vi "Swerve Open 2020.vi"(10 "Drive Current Limit":dbl=50.0 format="%#_13g", 11 "Enum":T2(ring)) -> ()   [LabVIEW 2018]
uses:
  <vilib>/Rock Robotics/WPI/ThirdParty/Phoenix-LabVIEW/Motor Controller/Controls/CTRE_Phoenix_MotorControl_FeedbackDevice.ctl
  <vilib>/Rock Robotics/WPI/ThirdParty/Phoenix-LabVIEW/Motor Controller/Controls/CTRE_Phoenix_MotorControl_NeutralMode.ctl
  <vilib>/Rock Robotics/WPI/ThirdParty/Phoenix-LabVIEW/Motor Controller/Get/CTRE_Phoenix_MotorController_GetPulseWidthAll.vi
  <vilib>/Rock Robotics/Network Tables/NT Write Numeric Array.vi
  <vilib>/Rock Robotics/Network Tables/NT Read Numeric Array.vi
panel:
  out "Sticky Faults 12":T1
  out "Sticky Faults 11":T1={"Under Voltage"=TRUE, "Forward Limit Switch"=FALSE, "Reverse Limit Switch"=FALSE, "Forward Soft Limit"=FALSE, "Reverse Soft Limit"=FALSE, "Reset During Enable"=FALSE, "Sensor Overflow"=FALSE, "Sensor Out of Phase"=FALSE, "Hardware ESD Reset"=FALSE, "Remote Loss of Signal"=FALSE}
  out "Sticky Faults 10":T1
  out "Sticky Faults 9":T1
  in  "Offsets":dbl[](array[numeric])=[5398.0, 5987.0, 35324.0, 34409.0]
  in  "Constants":T3={"P"=6.0, "I"=0.0, "D"=60.0, "F"=1.0, "Max Vel"=900.0, "Max Accel"=3000.0}
  # "Little Swerve"
  # "8"
  # "6"
  # "1210"
  # "FL"
  # "1909"
  # "2531"
  # "0"
  # "0"
  # "FR"
  # "1604"
  # "BL"
  # "40"
  # "80"
  # "BR"
  # "0.806"
  # "1.23"
  # "900"
  # "900"
  # "3600"
  # "3600"
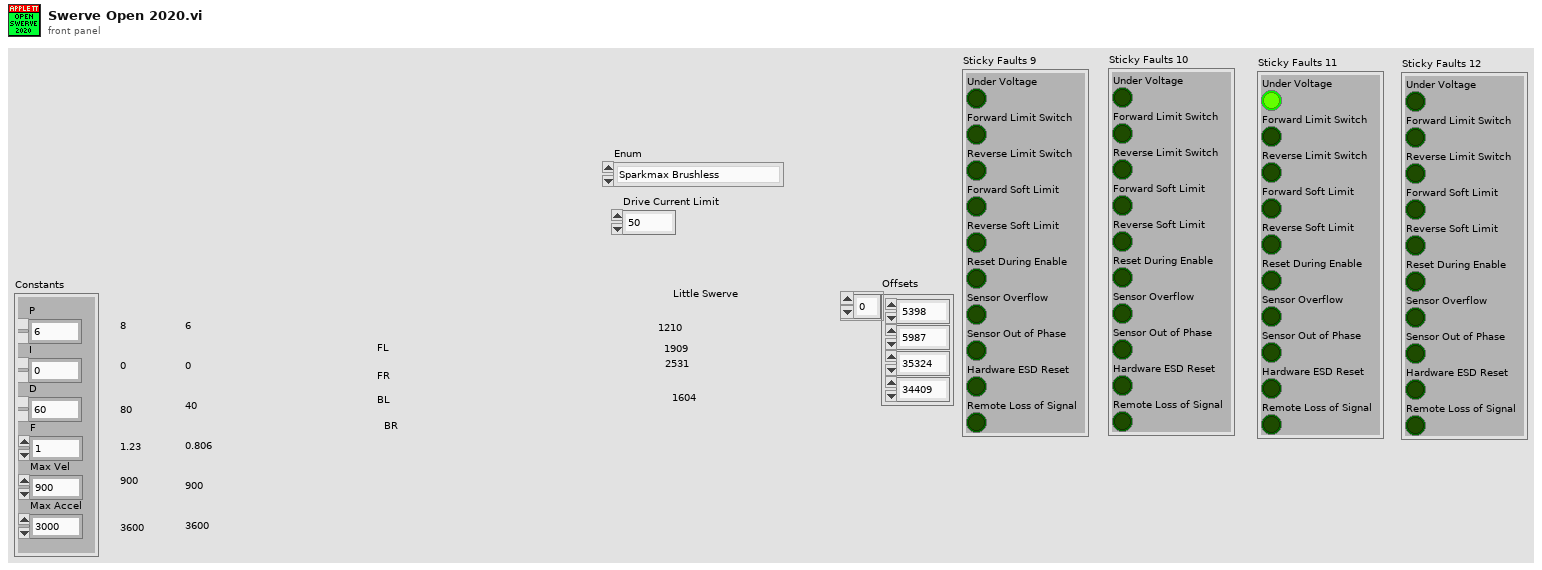
[diagram p1: front panel]
types:
  T1 = cluster{"Under Voltage":bool, "Forward Limit Switch":bool, "Reverse Limit Switch":bool, "Forward Soft Limit":bool, "Reverse Soft Limit":bool, "Reset During Enable":bool, "Sensor Overflow":bool, "Sensor Out of Phase":bool, "Hardware ESD Reset":bool, "Remote Loss of Signal":bool}
  T2 = enum16{"Sparkmax Brushless", "Talon SRX Brushed"}
  T3 = cluster{"P":dbl, "I":dbl, "D":dbl, "F":dbl, "Max Vel":dbl, "Max Accel":dbl}
  T4 = typedef "CTRE_Phoenix_MotorControl_NeutralMode.ctl" = enum8{"EEPROMSetting", "Override to Coast", "Override to Brake"}
  T5 = typedef "CTRE_Phoenix_MotorControl_FeedbackDevice.ctl" = i8
  T6 = typedef "WPI_MotorControlDeviceRef.ctl" = cluster{"DeviceStatus":errorcluster, "Type":T7, "PWM":cluster{"PWM Channel":T8, "DeadBand":T9}, "CAN":cluster{"Device Number":u8, "SetOutput VI Ref":variant, "GetOutput VI Ref":variant, "Enable VI Ref":variant, "Disable VI Ref":variant, "Data":variant}, "Invert":bool, "DIO PWM":cluster{"PWM \"Enable\" Channel":T8, "DIOChannel":T10, "PWM Rate":dbl}}
  T7 = typedef "WPI_MotorControlType.ctl" = enum16{"PWM", "CAN", "DIO PWM"}
  T8 = typedef "FPGA_DIOPWMChannel.ctl" = enum8{"PWM 0", "PWM 1", "PWM 2", "PWM 3", "PWM 4", "PWM 5", "PWM 6", "PWM 7", "PWM 8", "PWM 9", "PWM MXP 0", "PWM MXP 1", "PWM MXP 2", "PWM MXP 3", "PWM MXP 4", "PWM MXP 5", "PWM MXP 6", "PWM MXP 7", "PWM MXP 8", "PWM MXP 9", "Invalid"}
  T9 = typedef "WPI_PWMDeadband.ctl" = cluster{"Name":string, "maxPositivePwm":i32, "minPositivePwm":i32, "centerPwm":i32, "maxNegativePwm":i32, "minNegativePwm":i32, "angularRange":u16}
  T10 = typedef "FPGA_DIOChannel.ctl" = enum8{"DIO 0", "DIO 1", "DIO 2", "DIO 3", "DIO 4", "DIO 5", "DIO 6", "DIO 7", "DIO 8", "DIO 9", "DIO MXP 0", "DIO MXP 1", "DIO MXP 2", "DIO MXP 3", "DIO MXP 4", "DIO MXP 5", "DIO MXP 6", "DIO MXP 7", "DIO MXP 8", "DIO MXP 9", "DIO MXP 10", "DIO MXP 11", "DIO MXP 12", "DIO MXP 13", "DIO MXP 14", "DIO MXP 15", "SPI Port CS1", "SPI Port CS2", "SPI Port CS3", "SPI Port MISO", "SPI Port MOSI", "Invalid"}
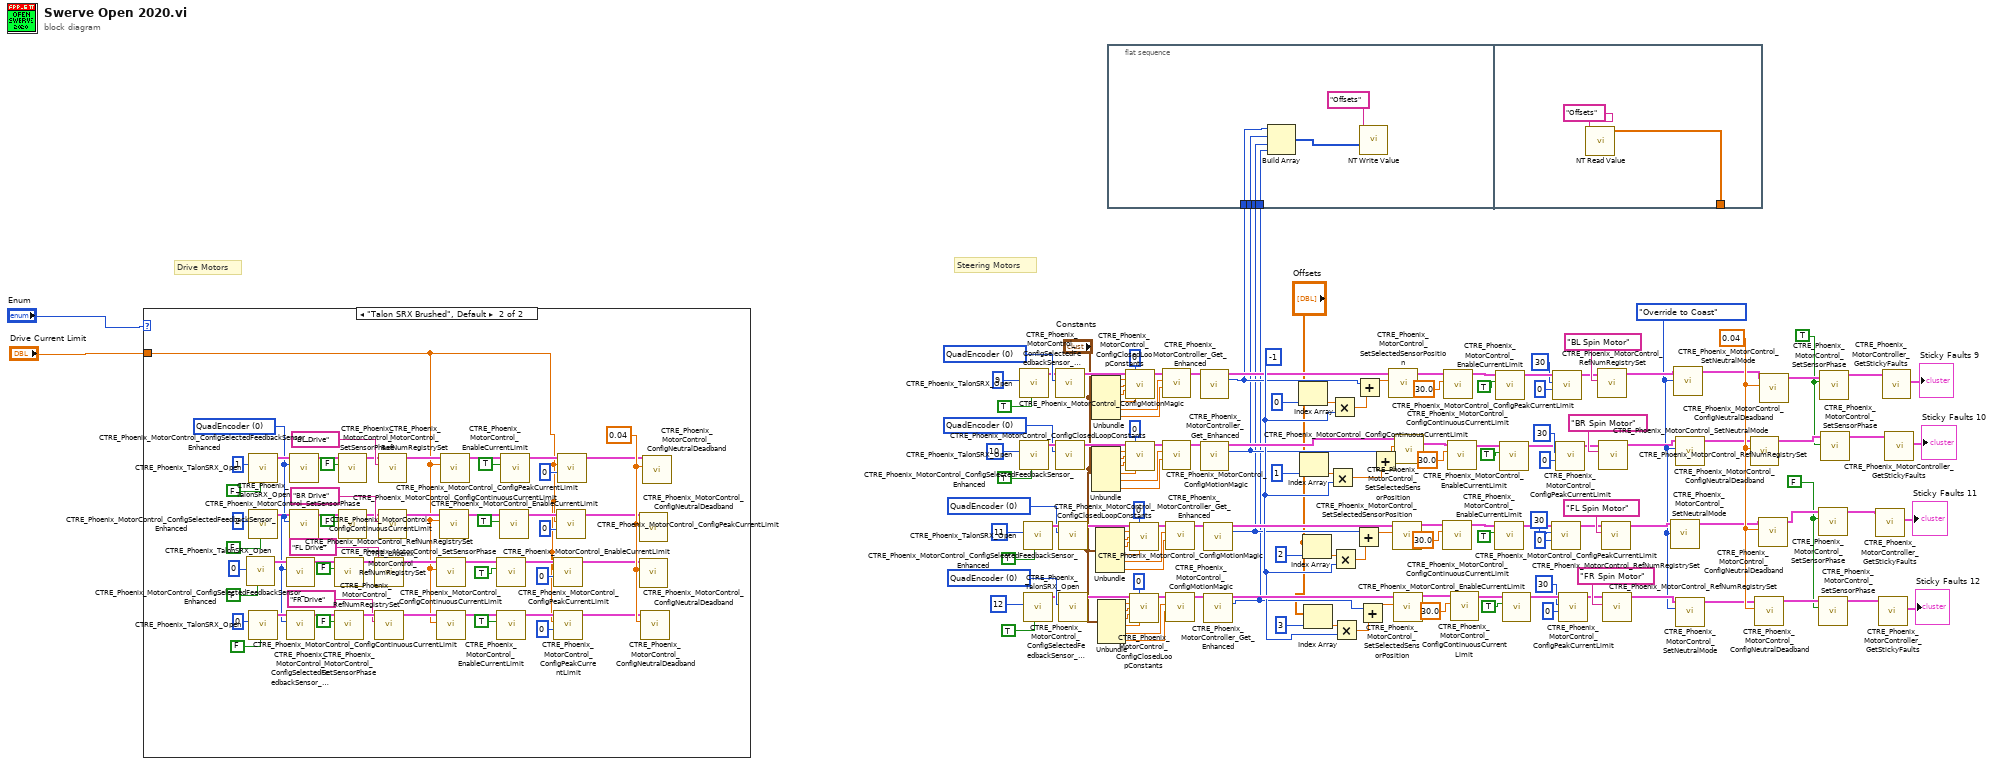
[diagram p0: block diagram]
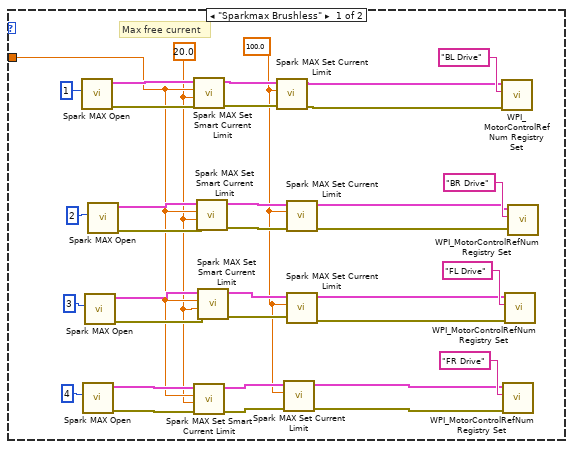
[diagram p2: hidden frame]
diagram:
  w10 = FALSE ("PhaseSensor")
  w11 = TRUE ("PhaseSensor")
  w32 = 0.04 ("Percent Deadband")
  w37 = CTRE_Phoenix_MotorControl_NeutralMode."Override to Coast" ("Motor Control Neutral Mode")
  w99 = T5 0 items=["None"=-1, "QuadEncoder"=0, "Analog"=2, "Tachometer"=4, "Pulse Width Encoded Position"=8, "Sensor Sum (S0 + S1)"=9, "Sensor Difference (D0 - D1)"=10, "Remote Source 0"=11, "Remote Source 1"=12, "Software Emulated"=15] ("Feedback Device")
  w100 = T5 0 items=["None"=-1, "QuadEncoder"=0, "Analog"=2, "Tachometer"=4, "Pulse Width Encoded Position"=8, "Sensor Sum (S0 + S1)"=9, "Sensor Difference (D0 - D1)"=10, "Remote Source 0"=11, "Remote Source 1"=12, "Software Emulated"=15] ("Feedback Device")
  w134 = T5 0 items=["None"=-1, "QuadEncoder"=0, "Analog"=2, "Tachometer"=4, "Pulse Width Encoded Position"=8, "Sensor Sum (S0 + S1)"=9, "Sensor Difference (D0 - D1)"=10, "Remote Source 0"=11, "Remote Source 1"=12, "Software Emulated"=15] ("Feedback Device")
  w133 = T5 0 items=["None"=-1, "QuadEncoder"=0, "Analog"=2, "Tachometer"=4, "Pulse Width Encoded Position"=8, "Sensor Sum (S0 + S1)"=9, "Sensor Difference (D0 - D1)"=10, "Remote Source 0"=11, "Remote Source 1"=12, "Software Emulated"=15] ("Feedback Device")
  w78 = -1 ("y")
  # "Steering Motors"
  # "Drive Motors"
  n1 = case shown="\"Talon SRX Brushed\", Default" "Enum" {
    tunnel: "Drive Current Limit" -> [w148 w181]
    frame "Sparkmax Brushless" {
      w146 = 20.0 ("Free Speed Current Limit (20A)")
      w147 = sgl 100.0 ("Current Limit A (100)")
      # "Max free current"
      n2 = call <vilib>:"Spark MAX Open.vi"("Device Number"=u8 1) -> ("error out"=w169:errorcluster, "MotorControlDeviceRef"=w168:T6)  [unwired: 9 in]
      n3 = call <vilib>:"Spark MAX Open.vi"("Device Number"=u8 4) -> ("error out"=w151:errorcluster, "MotorControlDeviceRef"=w152:T6)  [unwired: 9 in]
      n4 = call <vilib>:"Spark MAX Open.vi"("Device Number"=u8 3) -> ("error out"=w160:errorcluster, "MotorControlDeviceRef"=w161:T6)  [unwired: 9 in]
      n5 = call <vilib>:"Spark MAX Open.vi"("Device Number"=u8 2) -> ("error out"=w149:errorcluster, "MotorControlDeviceRef"=w150:T6)  [unwired: 9 in]
      n6 = call <vilib>:"Spark MAX Set Smart Current Limit.vi"("error in (no error)"=w169, "Free Speed Current Limit (20A)"=w146, "Primay Current Limit (80A)"=w148, "MotorControlDeviceRef in"=w168) -> ("error out"=w170:errorcluster, "MotorControlDeviceRef out"=w171:T6)  [unwired: 6 in]
      n7 = call <vilib>:"Spark MAX Set Smart Current Limit.vi"("error in (no error)"=w151, "Free Speed Current Limit (20A)"=w146, "Primay Current Limit (80A)"=w148, "MotorControlDeviceRef in"=w152) -> ("error out"=w162:errorcluster, "MotorControlDeviceRef out"=w163:T6)  [unwired: 6 in]
      n8 = call <vilib>:"Spark MAX Set Smart Current Limit.vi"("error in (no error)"=w149, "Free Speed Current Limit (20A)"=w146, "Primay Current Limit (80A)"=w148, "MotorControlDeviceRef in"=w150) -> ("error out"=w166:errorcluster, "MotorControlDeviceRef out"=w167:T6)  [unwired: 6 in]
      n9 = call <vilib>:"Spark MAX Set Smart Current Limit.vi"("error in (no error)"=w160, "Free Speed Current Limit (20A)"=w146, "Primay Current Limit (80A)"=w148, "MotorControlDeviceRef in"=w161) -> ("error out"=w164:errorcluster, "MotorControlDeviceRef out"=w165:T6)  [unwired: 6 in]
      n10 = call <vilib>:"Spark MAX Set Current Limit.vi"("error in (no error)"=w170, "Current Limit A (100)"=w147, "MotorControlDeviceRef in"=w171) -> ("error out"=w172:errorcluster, "MotorControlDeviceRef out"=w173:T6)  [unwired: 7 in]
      n11 = call <vilib>:"Spark MAX Set Current Limit.vi"("error in (no error)"=w162, "Current Limit A (100)"=w147, "MotorControlDeviceRef in"=w163) -> ("error out"=w153:errorcluster, "MotorControlDeviceRef out"=w154:T6)  [unwired: 7 in]
      n12 = call <vilib>:"Spark MAX Set Current Limit.vi"("error in (no error)"=w166, "Current Limit A (100)"=w147, "MotorControlDeviceRef in"=w167) -> ("error out"=w156:errorcluster, "MotorControlDeviceRef out"=w157:T6)  [unwired: 7 in]
      n13 = call <vilib>:"Spark MAX Set Current Limit.vi"("error in (no error)"=w164, "Current Limit A (100)"=w147, "MotorControlDeviceRef in"=w165) -> ("error out"=w158:errorcluster, "MotorControlDeviceRef out"=w159:T6)  [unwired: 7 in]
      n14 = call <vilib>:"WPI_MotorControlRefNum Registry Set.vi"("error in (no error)"=w172, "refnum name"="BL Drive", "MotorControlDevRef"=w173) -> ()  [unwired: 7 in, 2 out]
      n15 = call <vilib>:"WPI_MotorControlRefNum Registry Set.vi"("error in (no error)"=w153, "refnum name"="FR Drive", "MotorControlDevRef"=w154) -> ()  [unwired: 7 in, 2 out]
      n16 = call <vilib>:"WPI_MotorControlRefNum Registry Set.vi"("error in (no error)"=w158, "refnum name"="FL Drive", "MotorControlDevRef"=w159) -> ()  [unwired: 7 in, 2 out]
      n17 = call <vilib>:"WPI_MotorControlRefNum Registry Set.vi"("error in (no error)"=w156, "refnum name"="BR Drive", "MotorControlDevRef"=w157) -> ()  [unwired: 7 in, 2 out]
    }
    frame "Talon SRX Brushed", Default {
      w191 = 0.04 ("Percent Deadband")
      (unwired) u8 0 ("Device Number")
      (unwired) u8 0 ("Device Number")
      (unwired) u8 0 ("Device Number")
      (unwired) u8 0 ("Device Number")
      w192 = T5 0 items=["None"=-1, "QuadEncoder"=0, "Analog"=2, "Tachometer"=4, "Pulse Width Encoded Position"=8, "Sensor Sum (S0 + S1)"=9, "Sensor Difference (D0 - D1)"=10, "Remote Source 0"=11, "Remote Source 1"=12, "Software Emulated"=15] ("Feedback Device")
      n18 = call <vilib>:"CTRE_Phoenix_TalonSRX_Open.vi"("Invert"=FALSE, "Device Number"=u8 3) -> ("CAN Talon SRX Ref"=w199:T6)  [unwired: 8 in, 1 out]
      n19 = call <vilib>:"CTRE_Phoenix_TalonSRX_Open.vi"("Invert"=FALSE, "Device Number"=u8 1) -> ("CAN Talon SRX Ref"=w230:T6)  [unwired: 8 in, 1 out]
      n20 = call <vilib>:"CTRE_Phoenix_TalonSRX_Open.vi"("Invert"=FALSE, "Device Number"=u8 2) -> ("CAN Talon SRX Ref"=w231:T6)  [unwired: 8 in, 1 out]
      n21 = call <vilib>:"CTRE_Phoenix_TalonSRX_Open.vi"("Invert"=FALSE, "Device Number"=u8 4) -> ("CAN Talon SRX Ref"=w203:T6)  [unwired: 8 in, 1 out]
      n22 = call <vilib>:"CTRE_Phoenix_MotorControl_ConfigSelectedFeedbackSensor_Enhanced.vi"("Feedback Device"=w192, "PhoenixMotorControlDevRef"=w199) -> ("PhoenixMotorControlDevRef"=w198:T6)  [unwired: 8 in, 1 out]
      n23 = call <vilib>:"CTRE_Phoenix_MotorControl_ConfigSelectedFeedbackSensor_Enhanced.vi"("Feedback Device"=w192, "PhoenixMotorControlDevRef"=w203) -> ("PhoenixMotorControlDevRef"=w205:T6)  [unwired: 8 in, 1 out]
      n24 = call <vilib>:"CTRE_Phoenix_MotorControl_ConfigSelectedFeedbackSensor_Enhanced.vi"("Feedback Device"=w192, "PhoenixMotorControlDevRef"=w230) -> ("PhoenixMotorControlDevRef"=w226:T6)  [unwired: 8 in, 1 out]
      n25 = call <vilib>:"CTRE_Phoenix_MotorControl_ConfigSelectedFeedbackSensor_Enhanced.vi"("Feedback Device"=w192, "PhoenixMotorControlDevRef"=w231) -> ("PhoenixMotorControlDevRef"=w229:T6)  [unwired: 8 in, 1 out]
      n26 = call <vilib>:"CTRE_Phoenix_MotorControl_SetSensorPhase.vi"("PhaseSensor"=FALSE, "PhoenixMotorControlDevRef"=w198) -> ("PhoenixMotorControlDevRef"=w197:T6)  [unwired: 8 in, 1 out]
      n27 = call <vilib>:"CTRE_Phoenix_MotorControl_SetSensorPhase.vi"("PhaseSensor"=FALSE, "PhoenixMotorControlDevRef"=w205) -> ("PhoenixMotorControlDevRef"=w204:T6)  [unwired: 8 in, 1 out]
      n28 = call <vilib>:"CTRE_Phoenix_MotorControl_SetSensorPhase.vi"("PhaseSensor"=FALSE, "PhoenixMotorControlDevRef"=w226) -> ("PhoenixMotorControlDevRef"=w227:T6)  [unwired: 8 in, 1 out]
      n29 = call <vilib>:"CTRE_Phoenix_MotorControl_SetSensorPhase.vi"("PhaseSensor"=FALSE, "PhoenixMotorControlDevRef"=w229) -> ("PhoenixMotorControlDevRef"=w228:T6)  [unwired: 8 in, 1 out]
      n30 = call <vilib>:"CTRE_Phoenix_MotorControl_RefNumRegistrySet.vi"("refnum name"="FL Drive", "PhoenixMotorControlDevRef"=w197) -> ("PhoenixMotorControlDevRef"=w196:T6)  [unwired: 8 in, 1 out]
      n31 = call <vilib>:"CTRE_Phoenix_MotorControl_RefNumRegistrySet.vi"("refnum name"="FR Drive", "PhoenixMotorControlDevRef"=w204) -> ("PhoenixMotorControlDevRef"=w213:T6)  [unwired: 8 in, 1 out]
      n32 = call <vilib>:"CTRE_Phoenix_MotorControl_RefNumRegistrySet.vi"("refnum name"="BL Drive", "PhoenixMotorControlDevRef"=w227) -> ("PhoenixMotorControlDevRef"=w214:T6)  [unwired: 8 in, 1 out]
      n33 = call <vilib>:"CTRE_Phoenix_MotorControl_RefNumRegistrySet.vi"("refnum name"="BR Drive", "PhoenixMotorControlDevRef"=w228) -> ("PhoenixMotorControlDevRef"=w219:T6)  [unwired: 8 in, 1 out]
      n34 = call <vilib>:"CTRE_Phoenix_MotorControl_ConfigContinuousCurrentLimit.vi"("Continuous Current Limit (Amps)"=w181, "PhoenixMotorControlDevRef"=w196) -> ("PhoenixMotorControlDevRef"=w195:T6)  [unwired: 8 in, 1 out]
      n35 = call <vilib>:"CTRE_Phoenix_MotorControl_ConfigContinuousCurrentLimit.vi"("Continuous Current Limit (Amps)"=w181, "PhoenixMotorControlDevRef"=w213) -> ("PhoenixMotorControlDevRef"=w208:T6)  [unwired: 8 in, 1 out]
      n36 = call <vilib>:"CTRE_Phoenix_MotorControl_ConfigContinuousCurrentLimit.vi"("Continuous Current Limit (Amps)"=w181, "PhoenixMotorControlDevRef"=w219) -> ("PhoenixMotorControlDevRef"=w223:T6)  [unwired: 8 in, 1 out]
      n37 = call <vilib>:"CTRE_Phoenix_MotorControl_ConfigContinuousCurrentLimit.vi"("Continuous Current Limit (Amps)"=w181, "PhoenixMotorControlDevRef"=w214) -> ("PhoenixMotorControlDevRef"=w215:T6)  [unwired: 8 in, 1 out]
      n38 = call <vilib>:"CTRE_Phoenix_MotorControl_EnableCurrentLimit.vi"("Enable Current Limit?"=TRUE, "PhoenixMotorControlDevRef"=w195) -> ("PhoenixMotorControlDevRef"=w194:T6)  [unwired: 8 in, 1 out]
      n39 = call <vilib>:"CTRE_Phoenix_MotorControl_EnableCurrentLimit.vi"("Enable Current Limit?"=TRUE, "PhoenixMotorControlDevRef"=w208) -> ("PhoenixMotorControlDevRef"=w211:T6)  [unwired: 8 in, 1 out]
      n40 = call <vilib>:"CTRE_Phoenix_MotorControl_EnableCurrentLimit.vi"("Enable Current Limit?"=TRUE, "PhoenixMotorControlDevRef"=w223) -> ("PhoenixMotorControlDevRef"=w220:T6)  [unwired: 8 in, 1 out]
      n41 = call <vilib>:"CTRE_Phoenix_MotorControl_EnableCurrentLimit.vi"("Enable Current Limit?"=TRUE, "PhoenixMotorControlDevRef"=w215) -> ("PhoenixMotorControlDevRef"=w218:T6)  [unwired: 8 in, 1 out]
      n42 = call <vilib>:"CTRE_Phoenix_MotorControl_ConfigPeakCurrentLimit.vi"("Peak Current Maximum Duration (ms)"=0, "Peak Current (Amps)"=w181, "PhoenixMotorControlDevRef"=w194) -> ("PhoenixMotorControlDevRef"=w184:T6)  [unwired: 7 in, 1 out]
      n43 = call <vilib>:"CTRE_Phoenix_MotorControl_ConfigPeakCurrentLimit.vi"("Peak Current Maximum Duration (ms)"=0, "Peak Current (Amps)"=w181, "PhoenixMotorControlDevRef"=w211) -> ("PhoenixMotorControlDevRef"=w183:T6)  [unwired: 7 in, 1 out]
      n44 = call <vilib>:"CTRE_Phoenix_MotorControl_ConfigPeakCurrentLimit.vi"("Peak Current Maximum Duration (ms)"=0, "Peak Current (Amps)"=w181, "PhoenixMotorControlDevRef"=w220) -> ("PhoenixMotorControlDevRef"=w185:T6)  [unwired: 7 in, 1 out]
      n45 = call <vilib>:"CTRE_Phoenix_MotorControl_ConfigPeakCurrentLimit.vi"("Peak Current Maximum Duration (ms)"=0, "Peak Current (Amps)"=w181, "PhoenixMotorControlDevRef"=w218) -> ("PhoenixMotorControlDevRef"=w186:T6)  [unwired: 7 in, 1 out]
      n46 = call <vilib>:"CTRE_Phoenix_MotorControl_ConfigNeutralDeadband.vi"("Percent Deadband"=w191, "PhoenixMotorControlDevRef"=w185) -> ()  [unwired: 8 in, 2 out]
      n47 = call <vilib>:"CTRE_Phoenix_MotorControl_ConfigNeutralDeadband.vi"("Percent Deadband"=w191, "PhoenixMotorControlDevRef"=w184) -> ()  [unwired: 8 in, 2 out]
      n48 = call <vilib>:"CTRE_Phoenix_MotorControl_ConfigNeutralDeadband.vi"("Percent Deadband"=w191, "PhoenixMotorControlDevRef"=w183) -> ()  [unwired: 8 in, 2 out]
      n49 = call <vilib>:"CTRE_Phoenix_MotorControl_ConfigNeutralDeadband.vi"("Percent Deadband"=w191, "PhoenixMotorControlDevRef"=w186) -> ()  [unwired: 8 in, 2 out]
    }
  }
  n50 = call <vilib>:"CTRE_Phoenix_TalonSRX_Open.vi"("Invert"=TRUE, "Device Number"=u8 9) -> ("CAN Talon SRX Ref"=w123:T6)  [unwired: 8 in, 1 out]
  n51 = call <vilib>:"CTRE_Phoenix_TalonSRX_Open.vi"("Invert"=TRUE, "Device Number"=u8 10) -> ("CAN Talon SRX Ref"=w143:T6)  [unwired: 8 in, 1 out]
  n52 = call <vilib>:"CTRE_Phoenix_TalonSRX_Open.vi"("Invert"=TRUE, "Device Number"=u8 11) -> ("CAN Talon SRX Ref"=w110:T6)  [unwired: 8 in, 1 out]
  n53 = call <vilib>:"CTRE_Phoenix_TalonSRX_Open.vi"("Invert"=TRUE, "Device Number"=u8 12) -> ("CAN Talon SRX Ref"=w91:T6)  [unwired: 8 in, 1 out]
  n54 = call <vilib>:"CTRE_Phoenix_MotorControl_ConfigSelectedFeedbackSensor_Enhanced.vi"("Feedback Device"=w133, "PhoenixMotorControlDevRef"=w123) -> ("PhoenixMotorControlDevRef"=w126:T6)  [unwired: 8 in, 1 out]
  n55 = call <vilib>:"CTRE_Phoenix_MotorControl_ConfigSelectedFeedbackSensor_Enhanced.vi"("Feedback Device"=w134, "PhoenixMotorControlDevRef"=w143) -> ("PhoenixMotorControlDevRef"=w141:T6)  [unwired: 8 in, 1 out]
  n56 = call <vilib>:"CTRE_Phoenix_MotorControl_ConfigSelectedFeedbackSensor_Enhanced.vi"("Feedback Device"=w100, "PhoenixMotorControlDevRef"=w110) -> ("PhoenixMotorControlDevRef"=w107:T6)  [unwired: 8 in, 1 out]
  n57 = call <vilib>:"CTRE_Phoenix_MotorControl_ConfigSelectedFeedbackSensor_Enhanced.vi"("Feedback Device"=w99, "PhoenixMotorControlDevRef"=w91) -> ("PhoenixMotorControlDevRef"=w94:T6)  [unwired: 8 in, 1 out]
  n58 = Unbundle("Constants") -> ("P"=w127:dbl, "I"=w128:dbl, "D"=w129:dbl, "F"=w130:dbl, "Max Vel"=w131:dbl, "Max Accel"=w132:dbl)
  n59 = Unbundle("Constants") -> ("P"=w140:dbl, "I"=w139:dbl, "D"=w138:dbl, "F"=w137:dbl, "Max Vel"=w136:dbl, "Max Accel"=w135:dbl)
  n60 = Unbundle("Constants") -> ("P"=w106:dbl, "I"=w105:dbl, "D"=w104:dbl, "F"=w103:dbl, "Max Vel"=w102:dbl, "Max Accel"=w101:dbl)
  n61 = Unbundle("Constants") -> ("P"=w95:dbl, "I"=w96:dbl, "D"=w97:dbl, "F"=w98:dbl, "Max Vel"=w77:dbl, "Max Accel"=w76:dbl)
  n62 = flat-sequence {
    tunnel: w15 -> [w241]
    tunnel: w14 -> [w240]
    tunnel: w13 -> [w239]
    tunnel: w12 -> [w238]
    tunnel: [w242] -> _
    frame #0 {
      n63 = Build Array(w241, w240, w239, w238) -> (w236:i32[])
      n64 = call-poly <vilib>:"NT Write Value.vi"("Numeric Array"=w236, "Name"="Offsets") -> ()  [unwired: 9 in, 1 out]
    }
    frame #1 {
      n65 = call-poly <vilib>:"NT Read Value.vi"("Name"="Offsets") -> ("Numeric Array"=w242:dbl[])  [unwired: 9 in, 1 out]
    }
  }
  n66 = call <vilib>:"CTRE_Phoenix_MotorControl_ConfigClosedLoopConstants.vi"("PhoenixMotorControlDevRef"=w126, "slotIdx"=0, "P"=w127, "I"=w128, "D"=w129, "F"=w130) -> ("PhoenixMotorControlDevRef"=w125:T6)  [unwired: 8 in, 1 out]
  n67 = call <vilib>:"CTRE_Phoenix_MotorControl_ConfigClosedLoopConstants.vi"("PhoenixMotorControlDevRef"=w141, "slotIdx"=0, "P"=w140, "I"=w139, "D"=w138, "F"=w137) -> ("PhoenixMotorControlDevRef"=w142:T6)  [unwired: 8 in, 1 out]
  n68 = call <vilib>:"CTRE_Phoenix_MotorControl_ConfigClosedLoopConstants.vi"("PhoenixMotorControlDevRef"=w107, "slotIdx"=0, "P"=w106, "I"=w105, "D"=w104, "F"=w103) -> ("PhoenixMotorControlDevRef"=w108:T6)  [unwired: 8 in, 1 out]
  n69 = call <vilib>:"CTRE_Phoenix_MotorControl_ConfigClosedLoopConstants.vi"("PhoenixMotorControlDevRef"=w94, "slotIdx"=0, "P"=w95, "I"=w96, "D"=w97, "F"=w98) -> ("PhoenixMotorControlDevRef"=w93:T6)  [unwired: 8 in, 1 out]
  n70 = call <vilib>:"CTRE_Phoenix_MotorControl_ConfigMotionMagic.vi"("Acceleration"=w132, "Cruise Velocity"=w131, "PhoenixMotorControlDevRef"=w125) -> ("PhoenixMotorControlDevRef"=w124:T6)  [unwired: 7 in, 1 out]
  n71 = call <vilib>:"CTRE_Phoenix_MotorControl_ConfigMotionMagic.vi"("Acceleration"=w135, "Cruise Velocity"=w136, "PhoenixMotorControlDevRef"=w142) -> ("PhoenixMotorControlDevRef"=w111:T6)  [unwired: 7 in, 1 out]
  n72 = call <vilib>:"CTRE_Phoenix_MotorControl_ConfigMotionMagic.vi"("Acceleration"=w101, "Cruise Velocity"=w102, "PhoenixMotorControlDevRef"=w108) -> ("PhoenixMotorControlDevRef"=w109:T6)  [unwired: 7 in, 1 out]
  n73 = call <vilib>:"CTRE_Phoenix_MotorControl_ConfigMotionMagic.vi"("Acceleration"=w76, "Cruise Velocity"=w77, "PhoenixMotorControlDevRef"=w93) -> ("PhoenixMotorControlDevRef"=w92:T6)  [unwired: 7 in, 1 out]
  n74 = call-poly <vilib>:"CTRE_Phoenix_MotorController_Get_Enhanced.vi"("PhoenixMotorControlDevRef"=w124) -> ("PhoenixMotorControlDevRef"=w16:T6, "Pulse Width Position"=w15:i32)  [unwired: 9 in, 4 out]
  n75 = call-poly <vilib>:"CTRE_Phoenix_MotorController_Get_Enhanced.vi"("PhoenixMotorControlDevRef"=w111) -> ("PhoenixMotorControlDevRef"=w114:T6, "Pulse Width Position"=w14:i32)  [unwired: 9 in, 4 out]
  n76 = call-poly <vilib>:"CTRE_Phoenix_MotorController_Get_Enhanced.vi"("PhoenixMotorControlDevRef"=w109) -> ("PhoenixMotorControlDevRef"=w82:T6, "Pulse Width Position"=w13:i32)  [unwired: 9 in, 4 out]
  n77 = call-poly <vilib>:"CTRE_Phoenix_MotorController_Get_Enhanced.vi"("PhoenixMotorControlDevRef"=w92) -> ("PhoenixMotorControlDevRef"=w85:T6, "Pulse Width Position"=w12:i32)  [unwired: 9 in, 4 out]
  n78 = Index Array(array="Offsets", index=0) -> (element=w36:dbl)
  n79 = Index Array(array="Offsets", index=1) -> (element=w35:dbl)
  n80 = Index Array(array="Offsets", index=2) -> (element=w34:dbl)
  n81 = Index Array(array="Offsets", index=3) -> (element=w33:dbl)
  n82 = Multiply(x=w35, y=w78) -> (x*y=w115:dbl)
  n83 = Multiply(x=w36, y=w78) -> (x*y=w21:dbl)
  n84 = Multiply(x=w34, y=w78) -> (x*y=w22:dbl)
  n85 = Multiply(x=w33, y=w78) -> (x*y=w23:dbl)
  n86 = Add(x=w13, y=w22) -> (x+y=w18:dbl)
  n87 = Add(x=w15, y=w21) -> (x+y=w20:dbl)
  n88 = Add(x=w12, y=w23) -> (x+y=w17:dbl)
  n89 = Add(x=w14, y=w115) -> (x+y=w19:dbl)
  n90 = call <vilib>:"CTRE_Phoenix_MotorControl_SetSelectedSensorPosition.vi"("New Sensor Position"=w20, "PhoenixMotorControlDevRef"=w16) -> ("PhoenixMotorControlDevRef"=w51:T6)  [unwired: 8 in, 1 out]
  n91 = call <vilib>:"CTRE_Phoenix_MotorControl_SetSelectedSensorPosition.vi"("New Sensor Position"=w18, "PhoenixMotorControlDevRef"=w82) -> ("PhoenixMotorControlDevRef"=w47:T6)  [unwired: 8 in, 1 out]
  n92 = call <vilib>:"CTRE_Phoenix_MotorControl_SetSelectedSensorPosition.vi"("New Sensor Position"=w17, "PhoenixMotorControlDevRef"=w85) -> ("PhoenixMotorControlDevRef"=w48:T6)  [unwired: 8 in, 1 out]
  n93 = call <vilib>:"CTRE_Phoenix_MotorControl_SetSelectedSensorPosition.vi"("New Sensor Position"=w19, "PhoenixMotorControlDevRef"=w114) -> ("PhoenixMotorControlDevRef"=w50:T6)  [unwired: 8 in, 1 out]
  n94 = call <vilib>:"CTRE_Phoenix_MotorControl_ConfigContinuousCurrentLimit.vi"("Continuous Current Limit (Amps)"=30.0, "PhoenixMotorControlDevRef"=w47) -> ("PhoenixMotorControlDevRef"=w54:T6)  [unwired: 8 in, 1 out]
  n95 = call <vilib>:"CTRE_Phoenix_MotorControl_ConfigContinuousCurrentLimit.vi"("Continuous Current Limit (Amps)"=30.0, "PhoenixMotorControlDevRef"=w51) -> ("PhoenixMotorControlDevRef"=w65:T6)  [unwired: 8 in, 1 out]
  n96 = call <vilib>:"CTRE_Phoenix_MotorControl_ConfigContinuousCurrentLimit.vi"("Continuous Current Limit (Amps)"=30.0, "PhoenixMotorControlDevRef"=w50) -> ("PhoenixMotorControlDevRef"=w74:T6)  [unwired: 8 in, 1 out]
  n97 = call <vilib>:"CTRE_Phoenix_MotorControl_ConfigContinuousCurrentLimit.vi"("Continuous Current Limit (Amps)"=30.0, "PhoenixMotorControlDevRef"=w48) -> ("PhoenixMotorControlDevRef"=w56:T6)  [unwired: 8 in, 1 out]
  n98 = call <vilib>:"CTRE_Phoenix_MotorControl_EnableCurrentLimit.vi"("Enable Current Limit?"=TRUE, "PhoenixMotorControlDevRef"=w54) -> ("PhoenixMotorControlDevRef"=w53:T6)  [unwired: 8 in, 1 out]
  n99 = call <vilib>:"CTRE_Phoenix_MotorControl_EnableCurrentLimit.vi"("Enable Current Limit?"=TRUE, "PhoenixMotorControlDevRef"=w65) -> ("PhoenixMotorControlDevRef"=w69:T6)  [unwired: 8 in, 1 out]
  n100 = call <vilib>:"CTRE_Phoenix_MotorControl_EnableCurrentLimit.vi"("Enable Current Limit?"=TRUE, "PhoenixMotorControlDevRef"=w74) -> ("PhoenixMotorControlDevRef"=w70:T6)  [unwired: 8 in, 1 out]
  n101 = call <vilib>:"CTRE_Phoenix_MotorControl_EnableCurrentLimit.vi"("Enable Current Limit?"=TRUE, "PhoenixMotorControlDevRef"=w56) -> ("PhoenixMotorControlDevRef"=w60:T6)  [unwired: 8 in, 1 out]
  n102 = call <vilib>:"CTRE_Phoenix_MotorControl_ConfigPeakCurrentLimit.vi"("Peak Current Maximum Duration (ms)"=0, "Peak Current (Amps)"=30, "PhoenixMotorControlDevRef"=w53) -> ("PhoenixMotorControlDevRef"=w43:T6)  [unwired: 7 in, 1 out]
  n103 = call <vilib>:"CTRE_Phoenix_MotorControl_ConfigPeakCurrentLimit.vi"("Peak Current Maximum Duration (ms)"=0, "Peak Current (Amps)"=30, "PhoenixMotorControlDevRef"=w69) -> ("PhoenixMotorControlDevRef"=w45:T6)  [unwired: 7 in, 1 out]
  n104 = call <vilib>:"CTRE_Phoenix_MotorControl_ConfigPeakCurrentLimit.vi"("Peak Current Maximum Duration (ms)"=0, "Peak Current (Amps)"=30, "PhoenixMotorControlDevRef"=w70) -> ("PhoenixMotorControlDevRef"=w44:T6)  [unwired: 7 in, 1 out]
  n105 = call <vilib>:"CTRE_Phoenix_MotorControl_ConfigPeakCurrentLimit.vi"("Peak Current Maximum Duration (ms)"=0, "Peak Current (Amps)"=30, "PhoenixMotorControlDevRef"=w60) -> ("PhoenixMotorControlDevRef"=w42:T6)  [unwired: 7 in, 1 out]
  n106 = call <vilib>:"CTRE_Phoenix_MotorControl_RefNumRegistrySet.vi"("refnum name"="BL Spin Motor", "PhoenixMotorControlDevRef"=w45) -> ("PhoenixMotorControlDevRef"=w41:T6)  [unwired: 8 in, 1 out]
  n107 = call <vilib>:"CTRE_Phoenix_MotorControl_RefNumRegistrySet.vi"("refnum name"="BR Spin Motor", "PhoenixMotorControlDevRef"=w44) -> ("PhoenixMotorControlDevRef"=w40:T6)  [unwired: 8 in, 1 out]
  n108 = call <vilib>:"CTRE_Phoenix_MotorControl_RefNumRegistrySet.vi"("refnum name"="FL Spin Motor", "PhoenixMotorControlDevRef"=w43) -> ("PhoenixMotorControlDevRef"=w39:T6)  [unwired: 8 in, 1 out]
  n109 = call <vilib>:"CTRE_Phoenix_MotorControl_RefNumRegistrySet.vi"("refnum name"="FR Spin Motor", "PhoenixMotorControlDevRef"=w42) -> ("PhoenixMotorControlDevRef"=w38:T6)  [unwired: 8 in, 1 out]
  n110 = call <vilib>:"CTRE_Phoenix_MotorControl_SetNeutralMode.vi"("Motor Control Neutral Mode"=w37, "PhoenixMotorControlDevRef"=w39) -> ("PhoenixMotorControlDevRef"=w29:T6)  [unwired: 8 in, 1 out]
  n111 = call <vilib>:"CTRE_Phoenix_MotorControl_SetNeutralMode.vi"("Motor Control Neutral Mode"=w37, "PhoenixMotorControlDevRef"=w41) -> ("PhoenixMotorControlDevRef"=w31:T6)  [unwired: 8 in, 1 out]
  n112 = call <vilib>:"CTRE_Phoenix_MotorControl_SetNeutralMode.vi"("Motor Control Neutral Mode"=w37, "PhoenixMotorControlDevRef"=w40) -> ("PhoenixMotorControlDevRef"=w30:T6)  [unwired: 8 in, 1 out]
  n113 = call <vilib>:"CTRE_Phoenix_MotorControl_SetNeutralMode.vi"("Motor Control Neutral Mode"=w37, "PhoenixMotorControlDevRef"=w38) -> ("PhoenixMotorControlDevRef"=w28:T6)  [unwired: 8 in, 1 out]
  n114 = call <vilib>:"CTRE_Phoenix_MotorControl_ConfigNeutralDeadband.vi"("Percent Deadband"=w32, "PhoenixMotorControlDevRef"=w30) -> ("PhoenixMotorControlDevRef"=w24:T6)  [unwired: 8 in, 1 out]
  n115 = call <vilib>:"CTRE_Phoenix_MotorControl_ConfigNeutralDeadband.vi"("Percent Deadband"=w32, "PhoenixMotorControlDevRef"=w28) -> ("PhoenixMotorControlDevRef"=w25:T6)  [unwired: 8 in, 1 out]
  n116 = call <vilib>:"CTRE_Phoenix_MotorControl_ConfigNeutralDeadband.vi"("Percent Deadband"=w32, "PhoenixMotorControlDevRef"=w29) -> ("PhoenixMotorControlDevRef"=w26:T6)  [unwired: 8 in, 1 out]
  n117 = call <vilib>:"CTRE_Phoenix_MotorControl_ConfigNeutralDeadband.vi"("Percent Deadband"=w32, "PhoenixMotorControlDevRef"=w31) -> ("PhoenixMotorControlDevRef"=w27:T6)  [unwired: 8 in, 1 out]
  n118 = call <vilib>:"CTRE_Phoenix_MotorControl_SetSensorPhase.vi"("PhaseSensor"=w10, "PhoenixMotorControlDevRef"=w26) -> ("PhoenixMotorControlDevRef"=w3:T6)  [unwired: 8 in, 1 out]
  n119 = call <vilib>:"CTRE_Phoenix_MotorControl_SetSensorPhase.vi"("PhaseSensor"=w10, "PhoenixMotorControlDevRef"=w25) -> ("PhoenixMotorControlDevRef"=w4:T6)  [unwired: 8 in, 1 out]
  n120 = call <vilib>:"CTRE_Phoenix_MotorControl_SetSensorPhase.vi"("PhaseSensor"=w11, "PhoenixMotorControlDevRef"=w27) -> ("PhoenixMotorControlDevRef"=w9:T6)  [unwired: 8 in, 1 out]
  n121 = call <vilib>:"CTRE_Phoenix_MotorControl_SetSensorPhase.vi"("PhaseSensor"=w11, "PhoenixMotorControlDevRef"=w24) -> ("PhoenixMotorControlDevRef"=w2:T6)  [unwired: 8 in, 1 out]
  n122 = call <vilib>:"CTRE_Phoenix_MotorController_GetStickyFaults.vi"("PhoenixMotorControlDevRef"=w3) -> ("Sticky Faults"=→"Sticky Faults 11":T1)  [unwired: 8 in, 2 out]
  n123 = call <vilib>:"CTRE_Phoenix_MotorController_GetStickyFaults.vi"("PhoenixMotorControlDevRef"=w4) -> ("Sticky Faults"=→"Sticky Faults 12":T1)  [unwired: 8 in, 2 out]
  n124 = call <vilib>:"CTRE_Phoenix_MotorController_GetStickyFaults.vi"("PhoenixMotorControlDevRef"=w9) -> ("Sticky Faults"=→"Sticky Faults 9":T1)  [unwired: 8 in, 2 out]
  n125 = call <vilib>:"CTRE_Phoenix_MotorController_GetStickyFaults.vi"("PhoenixMotorControlDevRef"=w2) -> ("Sticky Faults"=→"Sticky Faults 10":T1)  [unwired: 8 in, 2 out]
